vi "RQST Comm Lookup Table_Initialize.vi"(8 "error in (no error)":errorcluster) -> (0 "error out":errorcluster {"code" min=0 max=0}, 3 "vi reference":T1)   [LabVIEW 2015, in "J1939 Addon Engine.lvlib"]
uses:
  Engine/J1939 Addon Engine.lvlib
  Types/RQST Comm Lookup Table_Ref.ctl
  STM/Connection Manager/stm_ManagerStateVariables.ctl
  STM/TCP/stm_TCP Connection Info.ctl
  STM/_SubVIs/stm_MetaDataElement.ctl
  STM/Connection Manager/stm_TCPConnectionProperties.ctl
  STM/Connection Manager/stm_TCPConnectionMethod.ctl
  J1939 Addon Shared.lvlib
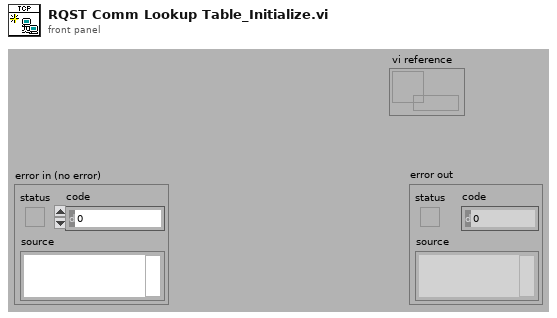
[diagram p1: front panel]
types:
  T1 = typedef "J1939 Addon Shared.lvlib/RQST Comm Lookup Table_Ref.ctl" = refnum<data-value>
  T2 = typedef "J1939 Addon Shared.lvlib/stm_ManagerStateVariables.ctl" = cluster{"All Connections":T3[], "All Properties":T5[]}
  T3 = typedef "J1939 Addon Shared.lvlib/stm_TCP Connection Info.ctl" = cluster{"connection ID":refnum<k5>, "Meta data":T4[]}
  T4 = typedef "J1939 Addon Shared.lvlib/stm_MetaDataElement.ctl" = string
  T5 = typedef "J1939 Addon Shared.lvlib/stm_TCPConnectionProperties.ctl" = cluster{"Name":string, "Address":string, "Custom":string}
  T6 = typedef "J1939 Addon Shared.lvlib/stm_TCPConnectionMethod.ctl" = enum16{"Initialize", "Add Connection", "Set Properties", "Get Connection(s)", "Remove Connection", "Remove All Connections", "Get Connection Count"}
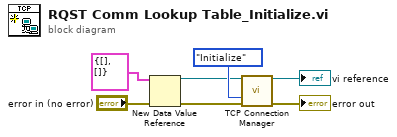
[diagram p0: block diagram]
diagram:
  n1 = New Data Value Reference(data value=T2 {"All Connections"=[], "All Properties"=[]}, error in="error in (no error)") -> (data value reference=w2:refnum<data-value>, error out=w5:errorcluster)
  n2 = call "TCP Connection Manager.vi"("TCP Ref"=w2, "Method"=stm_TCPConnectionMethod."Initialize", "error in (no error)"=w5) -> ("TCP Ref out"=→"vi reference":T1, "error out"=→"error out":errorcluster)  [unwired: 6 in, 5 out]
